vi "DrawRadarPlot.vi"(0 "reference in":refnum<class "LcWebView.lvclass">, 1 "XLabels":string[](array[string]), 2 "RadarPlot.Dataset":dbl[][](array[numeric]), 3 "RadarPlot.DatasetLabels":string[](array[string]), 5 "Error In":errorcluster, 6 "GenericPlotOptions":T1, 7 "BarPlot.PlotColours":u32[](array[numeric])) -> (14 "reference out":refnum<class "LcWebView.lvclass">, 19 "Error Out":errorcluster)   [LabVIEW 2021, in "LcWebView.lvclass"]
uses:
  LcWebView.lvclass
  ctrls/GenericPlotOption.ctl
  ctrls/LegendPosition.ctl
  cdfa7b6c-348e-4618-b79e-b8b55caa0d01.vi
  <vilib>/JDP Science/JSONtext/Variant to JSON Text.vi
  <vilib>/JDP Science/JSONtext/LVClass Serializer/JSONtext LVClass Serializer.lvclass
  LcWebView.lvclass/LcWebView.ctl
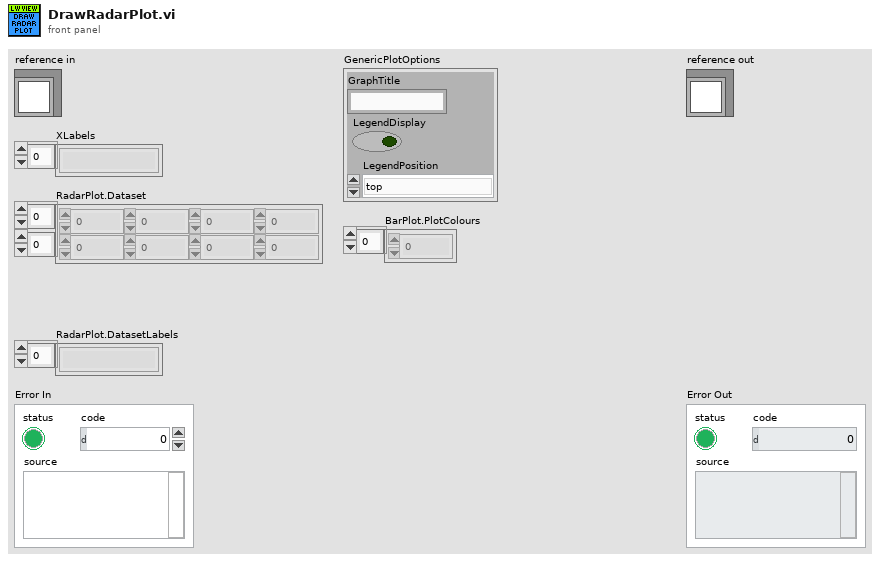
[diagram p1: front panel]
types:
  T1 = typedef "LcWebView.lvclass/GenericPlotOption.ctl" = cluster{"GraphTitle":string, "LegendDisplay":bool, "LegendPosition":T2}
  T2 = typedef "LcWebView.lvclass/LegendPosition.ctl" = enum16{"top", "right", "left", "bottom"}
  T3 = cluster{"action":string, "PlotData":string, "GenericPlotOptions":T1}
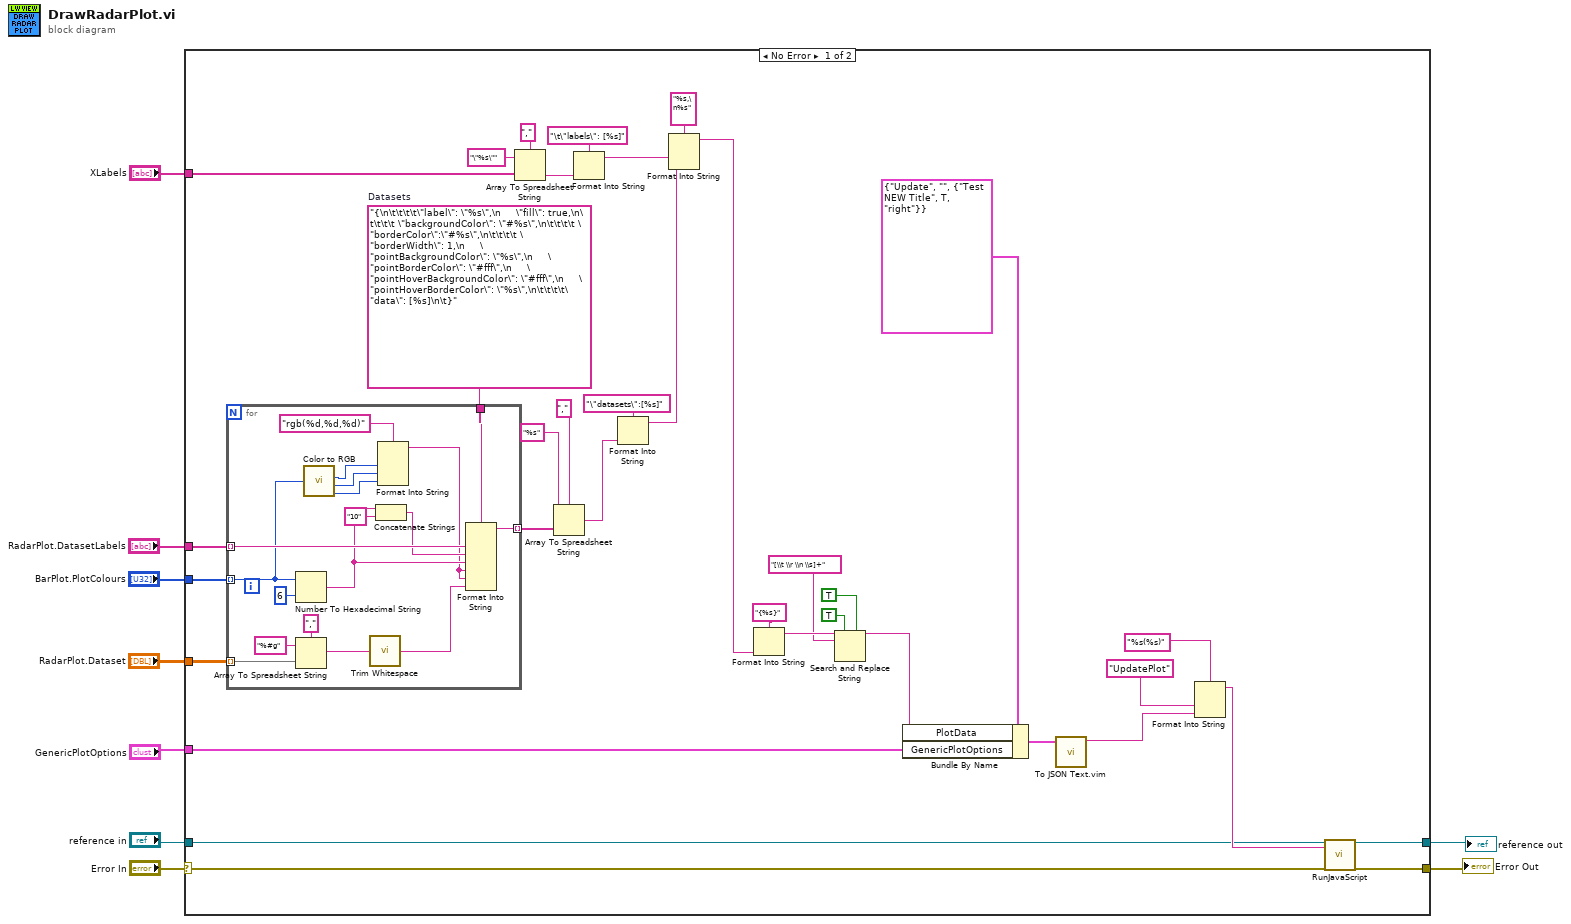
[diagram p0: block diagram]
diagram:
  n1 = case shown="No Error" "Error In" {
    selector: "Error In" -> [w14 w64]
    tunnel: [w15 w64] -> w1
    tunnel: [w16 w63] -> w2
    tunnel: "reference in" -> [w17 w63]
    tunnel: "RadarPlot.Dataset" -> [w35 _]
    tunnel: "BarPlot.PlotColours" -> [w34 _]
    tunnel: "RadarPlot.DatasetLabels" -> [w33 _]
    tunnel: "XLabels" -> [w32 _]
    tunnel: "GenericPlotOptions" -> [w24 _]
    frame No Error {
      w36 = "{\n\t\t\t\t\"label\": \"%s\",\n     \"fill\": true,\n\t\t\t\t \"backgroundColor\": \"#%s\",\n\t\t\t\t \"borderColor\":\"#%s\",\n\t\t\t\t \"borderWidth\": 1,\n     \"pointBackgroundColor\": \"%s\",\n     \"pointBorderColor\": \"#fff\",\n     \"pointHoverBackgroundColor\": \"#fff\",\n     \"pointHoverBorderColor\": \"%s\",\n\t\t\t\t\"data\": [%s]\n\t}"  # Datasets
      n2 = for {
        tunnel: w35 -> [w60] mode=indexing
        tunnel: w34 -> [w50] mode=indexing
        tunnel: w33 -> [w58] mode=indexing
        tunnel: [w57] -> w13 mode=indexing
        tunnel: w36 -> [w59]
        n3 = Number To Hexadecimal String(1:i16 6 ("width (-)"), 2:w50) -> (0:w53:string)
        n4 = Array To Spreadsheet String(delimiter (Tab)=",", array=w60, 3:"%#g" ("format string")) -> (spreadsheet string=w56:string)
        n5 = call <vilib>:"Color to RGB.vi"("Color"=w50) -> ("R"=w48:u8, "G"=w47:u8, "B"=w46:u8)  [unwired: 1 out]
        n6 = call <vilib>:"Trim Whitespace.vi"("string"=w56) -> ("trimmed string"=w54:string)  [unwired: 1 in]
        n7 = Concatenate Strings(w53, "10" ("string")) -> (w51:string)
        n8 = Format Into String(format string="rgb(%d,%d,%d)", w48, w47, w46) -> (resulting string=w45:string)  [unwired: 2 in, 1 out]
        n9 = Format Into String(format string=w59, w58, w51, w53, w45, w45, w54) -> (resulting string=w57:string)  [unwired: 2 in, 1 out]
      }
      n10 = Array To Spreadsheet String(delimiter (Tab)=",", array=w32, 3:"\"%s\"" ("format string")) -> (spreadsheet string=w40:string)
      n11 = Array To Spreadsheet String(delimiter (Tab)="," ("separator"), array=w13, 3:"%s" ("format string")) -> (spreadsheet string=w10:string)
      n12 = Format Into String(format string="\t\"labels\": [%s]", w40) -> (resulting string=w43:string)  [unwired: 2 in, 1 out]
      n13 = Format Into String(format string="\"datasets\":[%s]", w10) -> (resulting string=w38:string)  [unwired: 2 in, 1 out]
      n14 = Format Into String(format string="%s,\n%s", w43, w38) -> (resulting string=w30:string)  [unwired: 2 in, 1 out]
      n15 = Format Into String(format string="{%s}", w30) -> (resulting string=w29:string)  [unwired: 2 in, 1 out]
      n16 = Search and Replace String(replace all?=TRUE ("replace all? (F)"), multiline?=TRUE ("multiline? (F)"), input string=w29, search string="[\\t \\r \\n \\s]+") -> (result string=w28:string)  [unwired: 4 in, 3 out]
      n17 = Bundle By Name(cluster=T3 {"action"="Update", "PlotData"="", "GenericPlotOptions"={"GraphTitle"="Test NEW Title", "LegendDisplay"=TRUE, "LegendPosition"=enum."right"}}, "PlotData"=w28, "GenericPlotOptions"=w24) -> (w22:T3)
      n18 = call "To JSON Text.vim"("Anything"=w22) -> ("<JSON>"=w19:string)  [unwired: 9 in, 1 out]
      n19 = Format Into String(format string="%s(%s)", "UpdatePlot" ("input 1"), w19) -> (resulting string=w18:string)  [unwired: 2 in, 1 out]
      n20 = call-dynamic "RunJavaScript.vi"("reference in"=w17, "Java Script Function"=w18, "Error In"=w14) -> ("reference out"=w16:refnum<class "LcWebView.lvclass">, "Error Out"=w15:errorcluster)  [unwired: 13 in, 2 out]
    }
    frame Error {
    }
  }
  "Error Out" <- w1
  "reference out" <- w2
